vi "反控启动.vi"(10 "启动参数":T1(ring)=enum."CODCr", 11 "启动类型":T2(ring)) -> ()   [LabVIEW 2016]
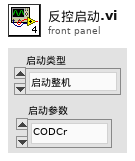
[diagram p1: front panel]
types:
  T1 = enum16{"未选择", "CODMn", "氨氮", "总磷", "总氮", "CODCr"}
  T2 = enum16{"启动整机", "停止整机", "标样核查", "加标回收", "平行样测试", "零点核查", "跨度核查", "校零", "校标"}
  T3 = cluster{"测量模式":enum16{"水样测量", "标样核查", "零点核查", "跨度核查", "空白测试", "加标回收", "平行样", "校零", "校标"}}
  T4 = cluster{"站号":u16, "量程切换":enum32{"H", "L", "AUTO"}, "控制命令":enum16{"启动测量", "标样核查", "零点核查", "跨度核查", "空白测试", "平行样测试", "加标回收", "空白校准", "标样校准", "初始化（清洗）", "停止测试", "仪器重启", "校时", "模式设置", "测量间隔设置"}, "模式设置":enum16{"待机", "连续模式", "周期模式", "定点模式", "受控模式", "手动模式"}, "测量间隔":u16}
  T5 = cluster{"status":bool, "代码":u16, "source":string}
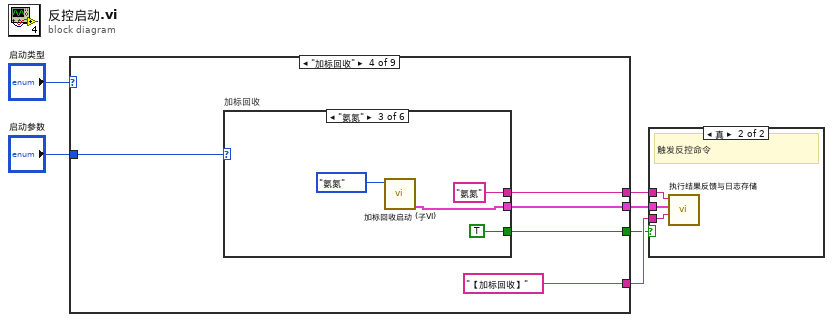
[diagram p0: block diagram]
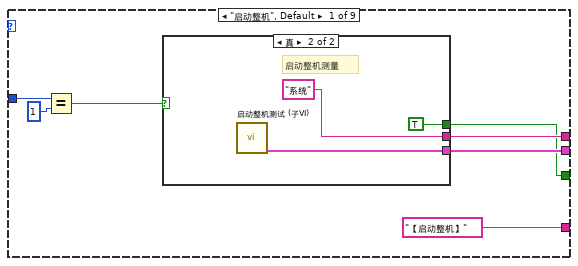
[diagram p3: hidden frame]
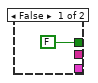
[diagram p4: hidden frame]
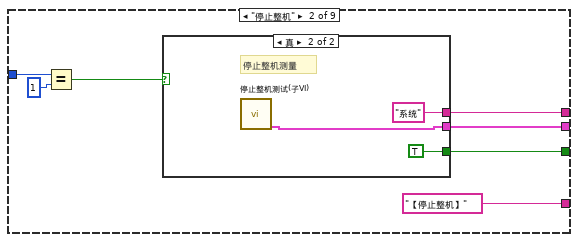
[diagram p5: hidden frame]
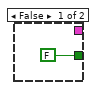
[diagram p6: hidden frame]
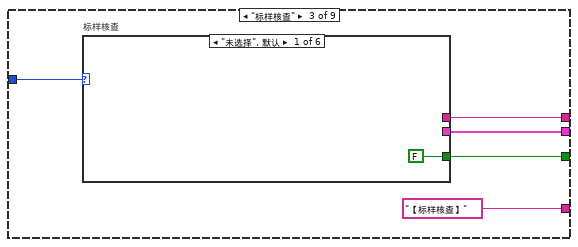
[diagram p7: hidden frame]
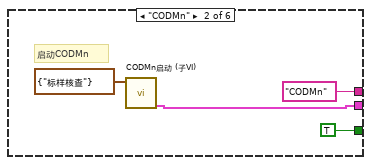
[diagram p8: hidden frame]
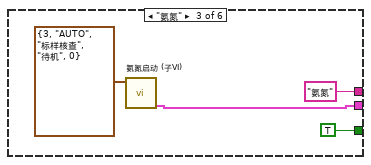
[diagram p9: hidden frame]
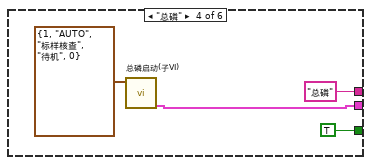
[diagram p10: hidden frame]
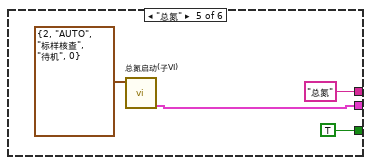
[diagram p11: hidden frame]
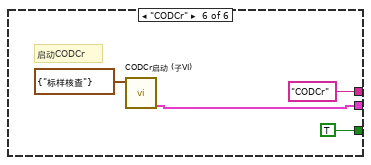
[diagram p12: hidden frame]
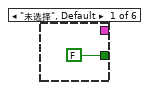
[diagram p13: hidden frame]
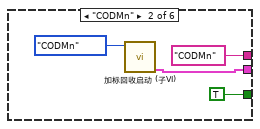
[diagram p14: hidden frame]
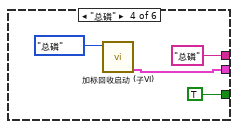
[diagram p15: hidden frame]
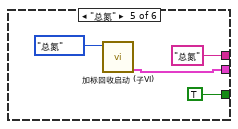
[diagram p16: hidden frame]
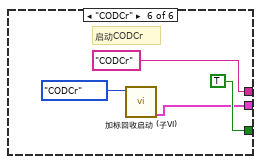
[diagram p17: hidden frame]
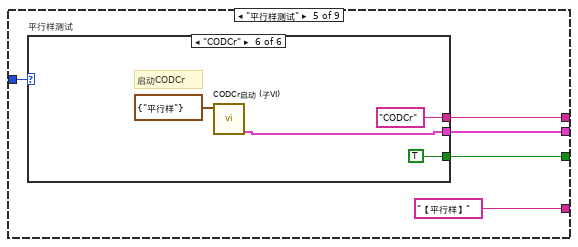
[diagram p18: hidden frame]
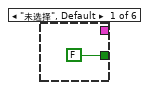
[diagram p19: hidden frame]
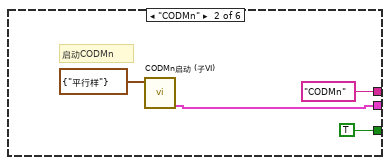
[diagram p20: hidden frame]
diagram:
  n1 = case shown="\"加标回收\"" "启动类型" {
    tunnel: "启动参数" -> [w13 w23 w33 w58 w85 w111 w137 w162 w189]
    tunnel: ["【启动整机】" ("日志信息") "【停止整机】" ("日志信息") "【标样核查】" ("日志信息") "【加标回收】" ("日志信息") "【平行样】" ("日志信息") "【零点核查】" ("日志信息") "【跨度核查】" ("日志信息") "【校零】" ("日志信息") "【校标】" ("日志信息")] -> w4
    tunnel: [w7 w19 w31 w56 w83 w108 w135 w160 w186] -> w3
    tunnel: [w10 w18 w30 w55 w82 w109 w134 w159 w187] -> w2
    tunnel: [w8 w20 w32 w57 w81 w107 w136 w161 w185] -> w1
    frame "启动整机", Default {
      n2 = Equal?(x=w13, y=1) -> (x = y?=w11:bool)
      n3 = case shown="真" w11 {
        tunnel: [_ w17] -> w10
        tunnel: [_ "系统" ("设备")] -> w8
        tunnel: [FALSE TRUE] -> w7
        frame False {
        }
        frame True {
          # "启动整机测量"
          n4 = call "启动整机测试 (子VI).vi"() -> ("error out"=w17:T5)  [unwired: 11 in]
        }
      }
    }
    frame "停止整机" {
      n5 = Equal?(x=w23, y=1) -> (x = y?=w22:bool)
      n6 = case shown="真" w22 {
        tunnel: [_ "系统" ("设备")] -> w20
        tunnel: [FALSE TRUE] -> w19
        tunnel: [_ w26] -> w18
        frame False {
        }
        frame True {
          # "停止整机测量"
          n7 = call "停止整机测试(子VI).vi"() -> ("error out"=w26:T5)  [unwired: 11 in]
        }
      }
    }
    frame "标样核查" {
      n8 = case "标样核查" shown="\"未选择\", 默认" w33 {
        tunnel: [_ "CODMn" ("设备") "氨氮" ("设备") "总磷" ("设备") "总氮" ("设备") "CODCr" ("设备")] -> w32
        tunnel: [_ w37 w41 w44 w48 w52] -> w30
        tunnel: [FALSE TRUE TRUE TRUE TRUE TRUE] -> w31
        frame "未选择", Default {
        }
        frame "CODMn" {
          # "启动CODMn"
          n9 = call "CODMn启动 (子VI).vi"("启动测量模式"=T3 {"测量模式"=enum."标样核查"}) -> ("error out"=w37:T5)  [unwired: 10 in]
        }
        frame "氨氮" {
          n10 = call "氨氮启动 (子VI).vi"("参数"=T4 {"站号"=3, "量程切换"=enum."AUTO", "控制命令"=enum."标样核查", "模式设置"=enum."待机", "测量间隔"=0}) -> ("error out"=w41:T5)  [unwired: 10 in]
        }
        frame "总磷" {
          n11 = call "总磷启动(子VI).vi"("参数"=T4 {"站号"=1, "量程切换"=enum."AUTO", "控制命令"=enum."标样核查", "模式设置"=enum."待机", "测量间隔"=0}) -> ("error out"=w44:T5)  [unwired: 10 in]
        }
        frame "总氮" {
          n12 = call "总氮启动(子VI).vi"("参数"=T4 {"站号"=2, "量程切换"=enum."AUTO", "控制命令"=enum."标样核查", "模式设置"=enum."待机", "测量间隔"=0}) -> ("error out"=w48:T5)  [unwired: 10 in]
        }
        frame "CODCr" {
          # "启动CODCr"
          n13 = call "CODCr启动 (子VI).vi"("启动测量模式"=T3 {"测量模式"=enum."标样核查"}) -> ("error out"=w52:T5)  [unwired: 10 in]
        }
      }
    }
    frame "加标回收" {
      n14 = case "加标回收" shown="\"氨氮\"" w58 {
        tunnel: [_ "CODMn" ("设备") "氨氮" ("设备") "总磷" ("设备") "总氮" ("设备") "CODCr" ("设备")] -> w57
        tunnel: [_ w61 w65 w69 w73 w77] -> w55
        tunnel: [FALSE TRUE TRUE TRUE TRUE TRUE] -> w56
        frame "未选择", Default {
        }
        frame "CODMn" {
          n15 = call "加标回收启动 (子VI).vi"("启动参数"=T1."CODMn") -> ("error out"=w61:T5)  [unwired: 10 in]
        }
        frame "氨氮" {
          n16 = call "加标回收启动 (子VI).vi"("启动参数"=T1."氨氮") -> ("error out"=w65:T5)  [unwired: 10 in]
        }
        frame "总磷" {
          n17 = call "加标回收启动 (子VI).vi"("启动参数"=T1."总磷") -> ("error out"=w69:T5)  [unwired: 10 in]
        }
        frame "总氮" {
          n18 = call "加标回收启动 (子VI).vi"("启动参数"=T1."总氮") -> ("error out"=w73:T5)  [unwired: 10 in]
        }
        frame "CODCr" {
          # "启动CODCr"
          n19 = call "加标回收启动 (子VI).vi"("启动参数"=T1."CODCr") -> ("error out"=w77:T5)  [unwired: 10 in]
        }
      }
    }
    frame "平行样测试" {
      n20 = case "平行样测试" shown="\"CODCr\"" w85 {
        tunnel: [_ "CODMn" ("设备") "氨氮" ("设备") "总磷" ("设备") "总氮" ("设备") "CODCr" ("设备")] -> w81
        tunnel: [_ w89 w93 w96 w100 w104] -> w82
        tunnel: [FALSE TRUE TRUE TRUE TRUE TRUE] -> w83
        frame "未选择", Default {
        }
        frame "CODMn" {
          # "启动CODMn"
          n21 = call "CODMn启动 (子VI).vi"("启动测量模式"=T3 {"测量模式"=enum."平行样"}) -> ("error out"=w89:T5)  [unwired: 10 in]
        }
        frame "氨氮" {
          n22 = call "氨氮启动 (子VI).vi"("参数"=T4 {"站号"=3, "量程切换"=enum."AUTO", "控制命令"=enum."平行样测试", "模式设置"=enum."待机", "测量间隔"=0}) -> ("error out"=w93:T5)  [unwired: 10 in]
        }
        frame "总磷" {
          n23 = call "总磷启动(子VI).vi"("参数"=T4 {"站号"=1, "量程切换"=enum."AUTO", "控制命令"=enum."平行样测试", "模式设置"=enum."待机", "测量间隔"=0}) -> ("error out"=w96:T5)  [unwired: 10 in]
        }
        frame "总氮" {
          n24 = call "总氮启动(子VI).vi"("参数"=T4 {"站号"=2, "量程切换"=enum."AUTO", "控制命令"=enum."平行样测试", "模式设置"=enum."待机", "测量间隔"=0}) -> ("error out"=w100:T5)  [unwired: 10 in]
        }
        frame "CODCr" {
          # "启动CODCr"
          n25 = call "CODCr启动 (子VI).vi"("启动测量模式"=T3 {"测量模式"=enum."平行样"}) -> ("error out"=w104:T5)  [unwired: 10 in]
        }
      }
    }
    frame "零点核查" {
      n26 = case "零点核查" shown="\"CODMn\"" w111 {
        tunnel: [_ "CODMn" ("设备") "氨氮" ("设备") "总磷" ("设备") "总氮" ("设备") "CODCr" ("设备")] -> w107
        tunnel: [_ w115 w119 w122 w126 w130] -> w109
        tunnel: [FALSE TRUE TRUE TRUE TRUE TRUE] -> w108
        frame "未选择", Default {
        }
        frame "CODMn" {
          # "启动CODMn"
          n27 = call "CODMn启动 (子VI).vi"("启动测量模式"=T3 {"测量模式"=enum."零点核查"}) -> ("error out"=w115:T5)  [unwired: 10 in]
        }
        frame "氨氮" {
          n28 = call "氨氮启动 (子VI).vi"("参数"=T4 {"站号"=3, "量程切换"=enum."AUTO", "控制命令"=enum."零点核查", "模式设置"=enum."待机", "测量间隔"=0}) -> ("error out"=w119:T5)  [unwired: 10 in]
        }
        frame "总磷" {
          n29 = call "总磷启动(子VI).vi"("参数"=T4 {"站号"=1, "量程切换"=enum."AUTO", "控制命令"=enum."零点核查", "模式设置"=enum."待机", "测量间隔"=0}) -> ("error out"=w122:T5)  [unwired: 10 in]
        }
        frame "总氮" {
          n30 = call "总氮启动(子VI).vi"("参数"=T4 {"站号"=2, "量程切换"=enum."AUTO", "控制命令"=enum."零点核查", "模式设置"=enum."待机", "测量间隔"=0}) -> ("error out"=w126:T5)  [unwired: 10 in]
        }
        frame "CODCr" {
          # "启动CODCr"
          n31 = call "CODCr启动 (子VI).vi"("启动测量模式"=T3 {"测量模式"=enum."零点核查"}) -> ("error out"=w130:T5)  [unwired: 10 in]
        }
      }
    }
    frame "跨度核查" {
      n32 = case "跨度核查" shown="\"CODMn\"" w137 {
        tunnel: [_ "CODMn" ("设备") "氨氮" ("设备") "总磷" ("设备") "总氮" ("设备") "CODCr" ("设备")] -> w136
        tunnel: [_ w141 w145 w148 w152 w156] -> w134
        tunnel: [FALSE TRUE TRUE TRUE TRUE TRUE] -> w135
        frame "未选择", Default {
        }
        frame "CODMn" {
          # "启动CODMn"
          n33 = call "CODMn启动 (子VI).vi"("启动测量模式"=T3 {"测量模式"=enum."跨度核查"}) -> ("error out"=w141:T5)  [unwired: 10 in]
        }
        frame "氨氮" {
          n34 = call "氨氮启动 (子VI).vi"("参数"=T4 {"站号"=3, "量程切换"=enum."AUTO", "控制命令"=enum."跨度核查", "模式设置"=enum."待机", "测量间隔"=0}) -> ("error out"=w145:T5)  [unwired: 10 in]
        }
        frame "总磷" {
          n35 = call "总磷启动(子VI).vi"("参数"=T4 {"站号"=1, "量程切换"=enum."AUTO", "控制命令"=enum."跨度核查", "模式设置"=enum."待机", "测量间隔"=0}) -> ("error out"=w148:T5)  [unwired: 10 in]
        }
        frame "总氮" {
          n36 = call "总氮启动(子VI).vi"("参数"=T4 {"站号"=2, "量程切换"=enum."AUTO", "控制命令"=enum."跨度核查", "模式设置"=enum."待机", "测量间隔"=0}) -> ("error out"=w152:T5)  [unwired: 10 in]
        }
        frame "CODCr" {
          # "启动CODCr"
          n37 = call "CODCr启动 (子VI).vi"("启动测量模式"=T3 {"测量模式"=enum."跨度核查"}) -> ("error out"=w156:T5)  [unwired: 10 in]
        }
      }
    }
    frame "校零" {
      n38 = case "校零" shown="\"CODMn\"" w162 {
        tunnel: [_ "CODMn" ("设备") "氨氮" ("设备") "总磷" ("设备") "总氮" ("设备") "CODCr" ("设备")] -> w161
        tunnel: [_ w167 w171 w174 w178 w182] -> w159
        tunnel: [FALSE TRUE TRUE TRUE TRUE TRUE] -> w160
        frame "未选择", Default {
        }
        frame "CODMn" {
          # "启动CODMn"
          n39 = call "CODMn启动 (子VI).vi"("启动测量模式"=T3 {"测量模式"=enum."校零"}) -> ("error out"=w167:T5)  [unwired: 10 in]
        }
        frame "氨氮" {
          n40 = call "氨氮启动 (子VI).vi"("参数"=T4 {"站号"=3, "量程切换"=enum."AUTO", "控制命令"=enum."空白校准", "模式设置"=enum."待机", "测量间隔"=0}) -> ("error out"=w171:T5)  [unwired: 10 in]
        }
        frame "总磷" {
          n41 = call "总磷启动(子VI).vi"("参数"=T4 {"站号"=1, "量程切换"=enum."AUTO", "控制命令"=enum."空白校准", "模式设置"=enum."待机", "测量间隔"=0}) -> ("error out"=w174:T5)  [unwired: 10 in]
        }
        frame "总氮" {
          n42 = call "总氮启动(子VI).vi"("参数"=T4 {"站号"=2, "量程切换"=enum."AUTO", "控制命令"=enum."空白校准", "模式设置"=enum."待机", "测量间隔"=0}) -> ("error out"=w178:T5)  [unwired: 10 in]
        }
        frame "CODCr" {
          # "启动CODCr"
          n43 = call "CODCr启动 (子VI).vi"("启动测量模式"=T3 {"测量模式"=enum."校零"}) -> ("error out"=w182:T5)  [unwired: 10 in]
        }
      }
    }
    frame "校标" {
      n44 = case "校标" shown="\"CODMn\"" w189 {
        tunnel: [_ "CODMn" ("设备") "氨氮" ("设备") "总磷" ("设备") "总氮" ("设备") "CODCr" ("设备")] -> w185
        tunnel: [_ w193 w197 w200 w204 w208] -> w187
        tunnel: [FALSE TRUE TRUE TRUE TRUE TRUE] -> w186
        frame "未选择", Default {
        }
        frame "CODMn" {
          # "启动CODMn"
          n45 = call "CODMn启动 (子VI).vi"("启动测量模式"=T3 {"测量模式"=enum."校标"}) -> ("error out"=w193:T5)  [unwired: 10 in]
        }
        frame "氨氮" {
          n46 = call "氨氮启动 (子VI).vi"("参数"=T4 {"站号"=3, "量程切换"=enum."AUTO", "控制命令"=enum."标样校准", "模式设置"=enum."待机", "测量间隔"=0}) -> ("error out"=w197:T5)  [unwired: 10 in]
        }
        frame "总磷" {
          n47 = call "总磷启动(子VI).vi"("参数"=T4 {"站号"=1, "量程切换"=enum."AUTO", "控制命令"=enum."标样校准", "模式设置"=enum."待机", "测量间隔"=0}) -> ("error out"=w200:T5)  [unwired: 10 in]
        }
        frame "总氮" {
          n48 = call "总氮启动(子VI).vi"("参数"=T4 {"站号"=2, "量程切换"=enum."AUTO", "控制命令"=enum."标样校准", "模式设置"=enum."待机", "测量间隔"=0}) -> ("error out"=w204:T5)  [unwired: 10 in]
        }
        frame "CODCr" {
          # "启动CODCr"
          n49 = call "CODCr启动 (子VI).vi"("启动测量模式"=T3 {"测量模式"=enum."校标"}) -> ("error out"=w208:T5)  [unwired: 10 in]
        }
      }
    }
  }
  n50 = case shown="真" w3 {
    tunnel: w4 -> [_ w211]
    tunnel: w2 -> [_ w212]
    tunnel: w1 -> [_ w213]
    frame False {
    }
    frame True {
      # "触发反控命令"
      n51 = call "执行结果反馈与日志存储.vi"("日志信息"=w211, "error out"=w212, "设备"=w213) -> ()  [unwired: 9 in]
    }
  }
